vi "Log Data to File.vi"(7 "WriteLogFile (T)":bool=TRUE, 8 "error in (no error)":errorcluster, 10 "Path":path) -> (0 "error out":errorcluster, 2 "Path out":path)   [LabVIEW 2020]
doc: "Developed by Kevin Thompson\nkevin@thompsonengineering.net\n\nCopyright 2018-2020\nThompson Engineering, LLC"
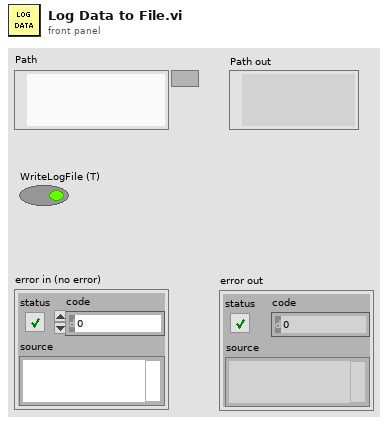
[diagram p1: front panel]
types:
  T1 = typedef "TD EventLogData--cluster.ctl" = cluster{"Timestamp":timestamp, "EventType":string, "EventData":string}
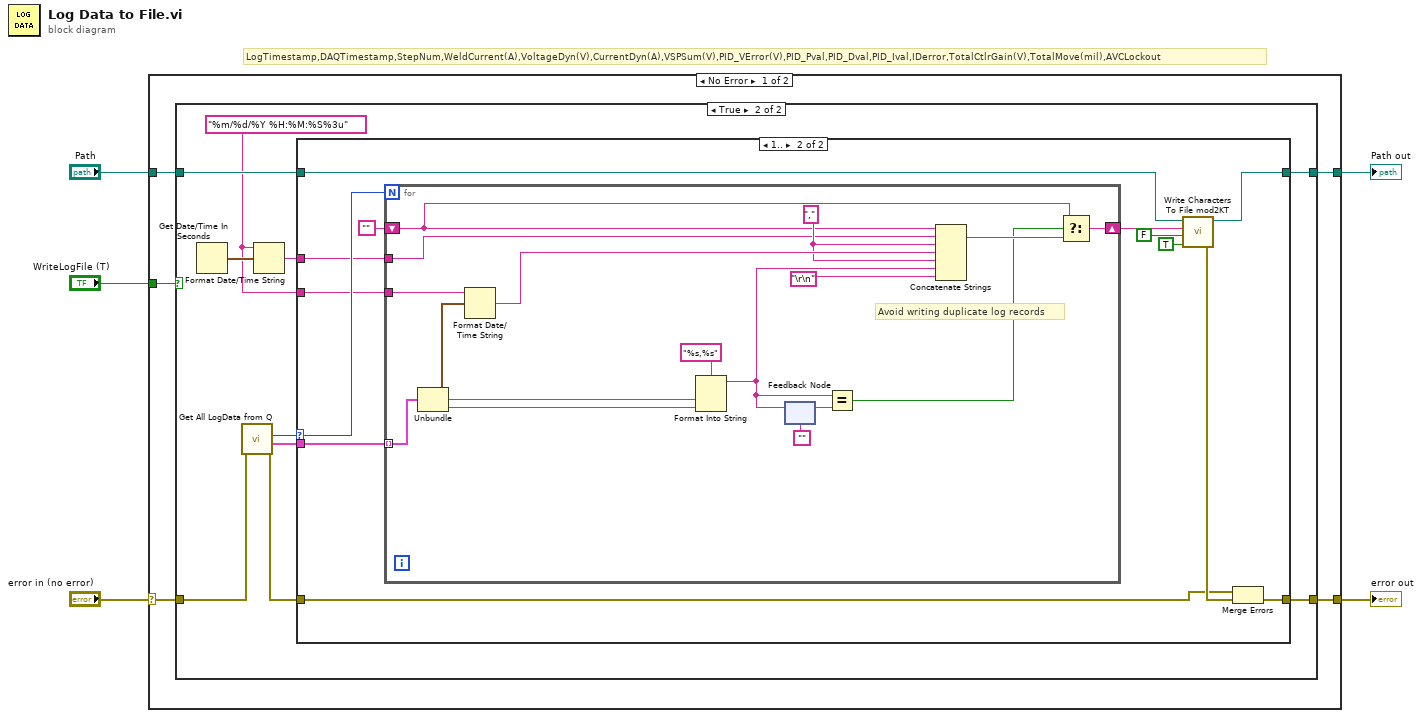
[diagram p0: block diagram]
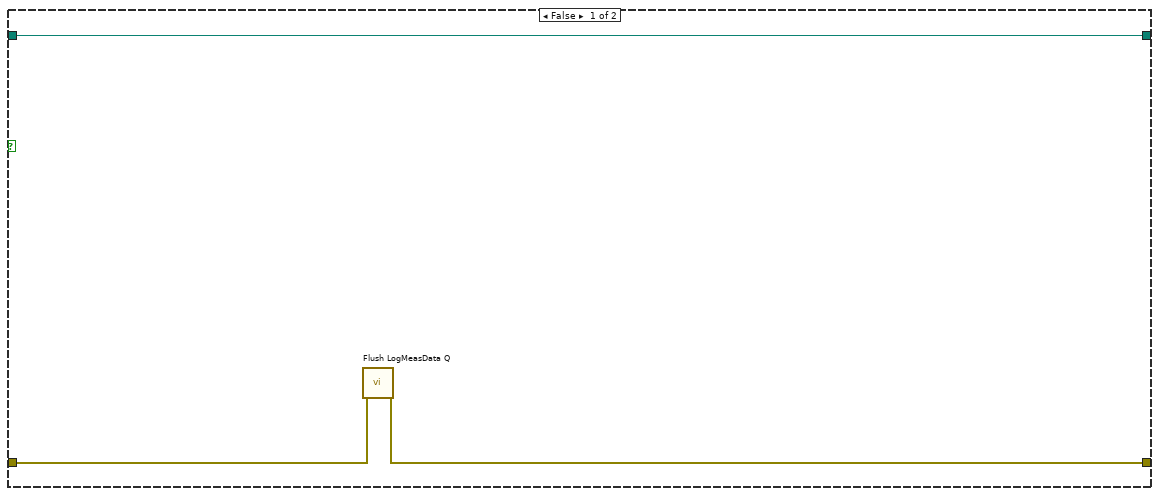
[diagram p2: hidden frame]
diagram:
  # "LogTimestamp,DAQTimestamp,StepNum,WeldCurrent(A),VoltageDyn(V),CurrentDyn(A),VSPSum(V),PID_VError(V),PID_Pval,PID_Dval,PID_Ival,IDerror,TotalCtlrGain(V),TotalMove(mil),AVCLockout"
  n1 = case shown="No Error" "error in (no error)" {
    selector: "error in (no error)" -> [w10 w57]
    tunnel: [w7 w57] -> w4
    tunnel: "Path" -> [w9 w56]
    tunnel: [w8 w56] -> w2
    tunnel: "WriteLogFile (T)" -> [w6 _]
    frame No Error {
      n2 = case shown="True" w6 {
        tunnel: w10 -> [w13 w17]
        tunnel: w9 -> [w11 w23]
        tunnel: [w11 w22] -> w8
        tunnel: [w12 w21] -> w7
        frame False {
          n3 = call "Flush LogMeasData Q.vi"("error in (no error)"=w13) -> ("error out"=w12:errorcluster)  [unwired: 8 in, 2 out]
        }
        frame True {
          w18 = "%m/%d/%Y %H:%M:%S%3u"
          n4 = Get Date/Time In Seconds() -> (seconds since 1Jan1904=w20:timestamp)
          n5 = call "Get All LogData from Q.vi"("error in (no error)"=w17) -> ("error out"=w16:errorcluster, "Events"=w14:T1[], "NumElements"=w15:i32)  [unwired: 7 in, 1 out]
          n6 = Format Date/Time String(time format string (%c)=w18, seconds (now)=w20) -> (date/time string=w19:string)  [unwired: 1 in]
          n7 = case shown="1.." w15 {
            selector: w15 -> [_ w38]
            tunnel: w14 -> [_ w37]
            tunnel: w23 -> [w25 w34]
            tunnel: [w25 w31] -> w22
            tunnel: [w24 w29] -> w21
            tunnel: w16 -> [w24 w28]
            tunnel: w19 -> [_ w27]
            tunnel: w18 -> [_ w26]
            frame ..0 {
            }
            frame 1.. {
              n8 = for {
                N: w38 -> [_]
                tunnel: w37 -> [w55] mode=indexing
                shift-right: [w43] -> w35
                shift-left: "" -> [w44]
                tunnel: w27 -> [w47]
                tunnel: w26 -> [w46]
                w49 = ","
                # "Avoid writing duplicate log records"
                n9 = Unbundle(w55) -> ("Timestamp"=w54:timestamp, "EventType"=w53:string, "EventData"=w52:string)
                n10 = Format Date/Time String(time format string (%c)=w46, seconds (now)=w54) -> (date/time string=w50:string)  [unwired: 1 in]
                n11 = Format Into String(format string="%s,%s", w53, w52) -> (resulting string=w40:string)  [unwired: 2 in, 1 out]
                n12 = feedback-in #1(w40) -> ()
                n13 = feedback #1("") -> (w41:string)
                n14 = Equal?(x=w40, y=w41) -> (x = y?=w39:bool)
                n15 = Concatenate Strings(w44, w47, w49, w50, w49, w40, "\r\n") -> (w45:string)
                n16 = Select(t=w44, s=w39, f=w45) -> (s? t:f=w43:string)
              }
              n17 = call <vilib>:"Write Characters To File mod2KT.vi"("append to file? (new file:F)"=TRUE, "advisory dialog? (display:T)"=FALSE, "character string"=w35, "file path (dialog if empty)"=w34) -> ("error out"=w30:errorcluster, "new file path (Not A Path if cancelled)"=w31:path)  [unwired: 2 in]
              n18 = Merge Errors(w28, w30) -> (w29:errorcluster)
            }
          }
        }
      }
    }
    frame Error {
    }
  }
  "error out" <- w4
  "Path out" <- w2
